vi "Gaussians model.vi"(3 "output control":T1, 4 "data":variant, 5 "X":dbl[](array[numeric]), 6 "a":dbl[](array[numeric])) -> (0 "error out":errorcluster, 1 "f'(X,a)":dbl[][](array[numeric]), 2 "f(X,a)":dbl[](array[numeric]))   [LabVIEW 2020]
doc: "Sum of three Gaussians, plus DC offset."
uses:
  <vilib>/gmath/NumericalOptimization/LM_output select.ctl
  <vilib>/gmath/NI_Gmath.lvlib
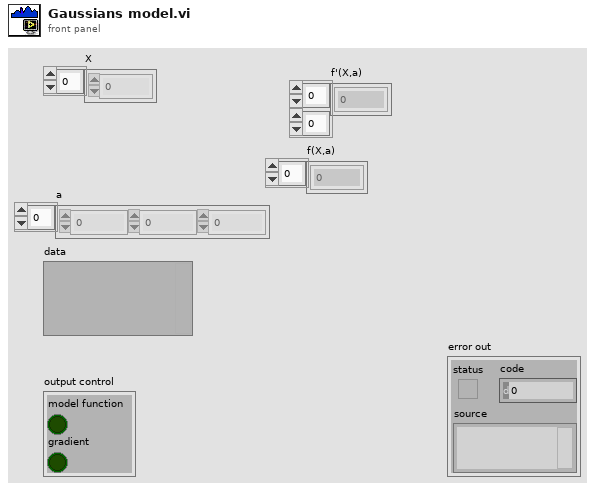
[diagram p1: front panel]
types:
  T1 = typedef "NI_Gmath.lvlib/LM_output select.ctl" = cluster{"model function":bool, "gradient":bool}
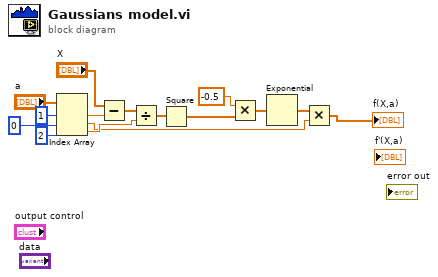
[diagram p0: block diagram]
diagram:
  n1 = Index Array(array="a", index #1=1 ("index"), index #2=0 ("index"), index #3=2 ("index")) -> (element #1=w13:dbl, element #2=w5:dbl, element #3=w11:dbl)
  n2 = Subtract(x="X", y=w13) -> (x-y=w12:dbl[])
  n3 = Divide(x=w12, y=w11) -> (x/y=w10:dbl[])
  n4 = Square(x=w10) -> (x^2=w9:dbl[])
  n5 = Multiply(x=-0.5, y=w9) -> (x*y=w7:dbl[])
  n6 = Exponential(1:w7) -> (0:w6:dbl[])
  n7 = Multiply(x=w6, y=w5) -> (x*y=→"f(X,a)":dbl[])
